vi "GageColorSubVI.vi"(11 "Numeric":dbl) -> (3 "Color Box":u32(colorbox))   [LabVIEW 2021]
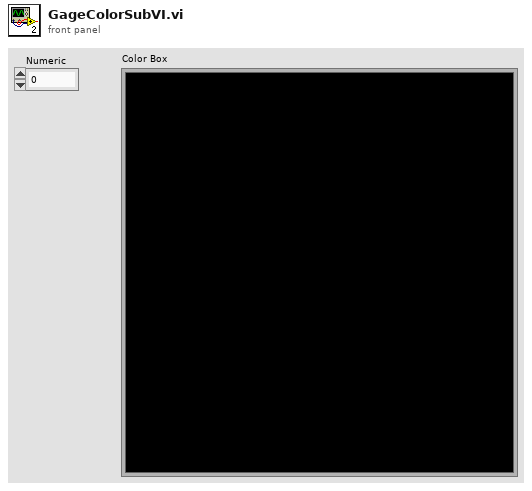
[diagram p1: front panel]
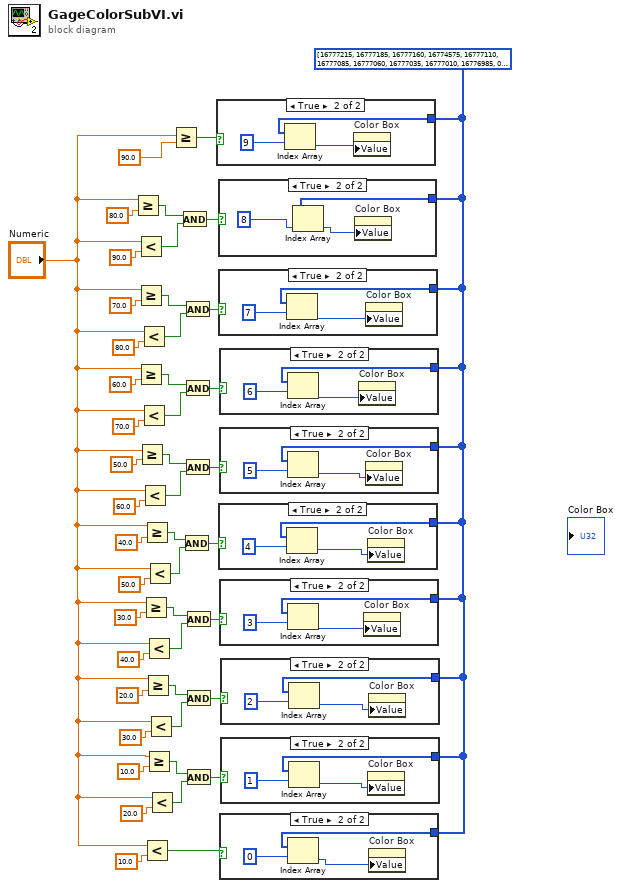
[diagram p0: block diagram]
diagram:
  w24 = u32[] [16777215, 16777185, 16777160, 16774575, 16777110, 16777085, 16777060, 16777035, 16777010, 16776985, 0, 0, 0, 16776960]
  n1 = Greater Or Equal?(x="Numeric", y=80.0) -> (x >= y?=w42:bool)
  n2 = Less?(x="Numeric", y=90.0) -> (x < y?=w40:bool)
  n3 = Greater Or Equal?(x="Numeric", y=70.0) -> (x >= y?=w38:bool)
  n4 = Greater Or Equal?(x="Numeric", y=60.0) -> (x >= y?=w34:bool)
  n5 = Greater Or Equal?(x="Numeric", y=50.0) -> (x >= y?=w1:bool)
  n6 = Less?(x="Numeric", y=80.0) -> (x < y?=w36:bool)
  n7 = Less?(x="Numeric", y=70.0) -> (x < y?=w32:bool)
  n8 = Less?(x="Numeric", y=60.0) -> (x < y?=w2:bool)
  n9 = Greater Or Equal?(x="Numeric", y=30.0) -> (x >= y?=w6:bool)
  n10 = Greater Or Equal?(x="Numeric", y=40.0) -> (x >= y?=w3:bool)
  n11 = Less?(x="Numeric", y=10.0) -> (x < y?=w12:bool)
  n12 = Greater Or Equal?(x="Numeric", y=20.0) -> (x >= y?=w8:bool)
  n13 = Less?(x="Numeric", y=40.0) -> (x < y?=w5:bool)
  n14 = Greater Or Equal?(x="Numeric", y=10.0) -> (x >= y?=w10:bool)
  n15 = Less?(x="Numeric", y=50.0) -> (x < y?=w4:bool)
  n16 = Less?(x="Numeric", y=30.0) -> (x < y?=w7:bool)
  n17 = Less?(x="Numeric", y=20.0) -> (x < y?=w9:bool)
  n18 = Greater Or Equal?(x="Numeric", y=90.0) -> (x >= y?=w46:bool)
  n19 = And(x=w42, y=w40) -> (x .and. y?=w43:bool)
  n20 = And(x=w3, y=w4) -> (x .and. y?=w28:bool)
  n21 = And(x=w38, y=w36) -> (x .and. y?=w30:bool)
  n22 = And(x=w34, y=w32) -> (x .and. y?=w31:bool)
  n23 = And(x=w1, y=w2) -> (x .and. y?=w29:bool)
  n24 = And(x=w6, y=w5) -> (x .and. y?=w26:bool)
  n25 = And(x=w8, y=w7) -> (x .and. y?=w27:bool)
  n26 = And(x=w10, y=w9) -> (x .and. y?=w25:bool)
  n27 = case shown="True" w46 {
    tunnel: w24 -> [_ w49]
    frame False {
    }
    frame True {
      n28 = Index Array(array=w49, index=9) -> (element=w47:u32)
      n29 = property on="Color Box" class="ColBox"("Value"=w47) -> ()  [unwired: 2 in, 2 out]
    }
  }
  n30 = case shown="True" w43 {
    tunnel: w24 -> [_ w52]
    frame False {
    }
    frame True {
      n31 = Index Array(array=w52, index=8) -> (element=w50:u32)
      n32 = property on="Color Box" class="ColBox"("Value"=w50) -> ()  [unwired: 2 in, 2 out]
    }
  }
  n33 = case shown="True" w30 {
    tunnel: w24 -> [_ w55]
    frame False {
    }
    frame True {
      n34 = Index Array(array=w55, index=7) -> (element=w53:u32)
      n35 = property on="Color Box" class="ColBox"("Value"=w53) -> ()  [unwired: 2 in, 2 out]
    }
  }
  n36 = case shown="True" w28 {
    tunnel: w24 -> [_ w58]
    frame False {
    }
    frame True {
      n37 = Index Array(array=w58, index=4) -> (element=w56:u32)
      n38 = property on="Color Box" class="ColBox"("Value"=w56) -> ()  [unwired: 2 in, 2 out]
    }
  }
  n39 = case shown="True" w31 {
    tunnel: w24 -> [_ w61]
    frame False {
    }
    frame True {
      n40 = Index Array(array=w61, index=6) -> (element=w59:u32)
      n41 = property on="Color Box" class="ColBox"("Value"=w59) -> ()  [unwired: 2 in, 2 out]
    }
  }
  n42 = case shown="True" w29 {
    tunnel: w24 -> [_ w64]
    frame False {
    }
    frame True {
      n43 = Index Array(array=w64, index=5) -> (element=w62:u32)
      n44 = property on="Color Box" class="ColBox"("Value"=w62) -> ()  [unwired: 2 in, 2 out]
    }
  }
  n45 = case shown="True" w26 {
    tunnel: w24 -> [_ w67]
    frame False {
    }
    frame True {
      n46 = Index Array(array=w67, index=3) -> (element=w65:u32)
      n47 = property on="Color Box" class="ColBox"("Value"=w65) -> ()  [unwired: 2 in, 2 out]
    }
  }
  n48 = case shown="True" w12 {
    tunnel: w24 -> [_ w70]
    frame False {
    }
    frame True {
      n49 = Index Array(array=w70, index=0) -> (element=w68:u32)
      n50 = property on="Color Box" class="ColBox"("Value"=w68) -> ()  [unwired: 2 in, 2 out]
    }
  }
  n51 = case shown="True" w27 {
    tunnel: w24 -> [_ w73]
    frame False {
    }
    frame True {
      n52 = Index Array(array=w73, index=2) -> (element=w71:u32)
      n53 = property on="Color Box" class="ColBox"("Value"=w71) -> ()  [unwired: 2 in, 2 out]
    }
  }
  n54 = case shown="True" w25 {
    tunnel: w24 -> [_ w76]
    frame False {
    }
    frame True {
      n55 = Index Array(array=w76, index=1) -> (element=w74:u32)
      n56 = property on="Color Box" class="ColBox"("Value"=w74) -> ()  [unwired: 2 in, 2 out]
    }
  }
